vi "sir_v2.vi"() -> ()   [LabVIEW 2009]
panel:
  in  "stop":bool
  out "Sir de caractere cu majuscule":string="APLICATIE LABWIEW\n"
  in  "Sir de caractere cu majuscule si minuscule":string="Aplicatie LabWIEW\n"
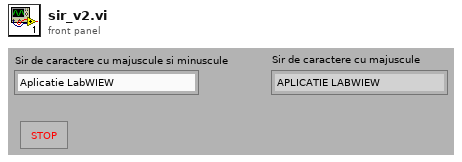
[diagram p1: front panel]
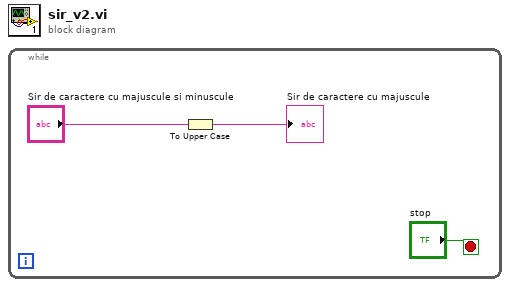
[diagram p0: block diagram]
diagram:
  n1 = while {
    stop <- "stop" stop-if-true
    n2 = To Upper Case(1:"Sir de caractere cu majuscule si minuscule") -> (0:→"Sir de caractere cu majuscule":string)
  }
